vi "NFC_Connect.vi"(9 "VISA resource name":refnum<visa-resource-name>="COM1") -> (1 "NFC":bool, 2 "Response":string)   [LabVIEW 2017]
uses:
  Ctrls/Serial_Settings.ctl
  <vilib>/Instr/_visa.llb/VISA Configure Serial Port (Instr).vi
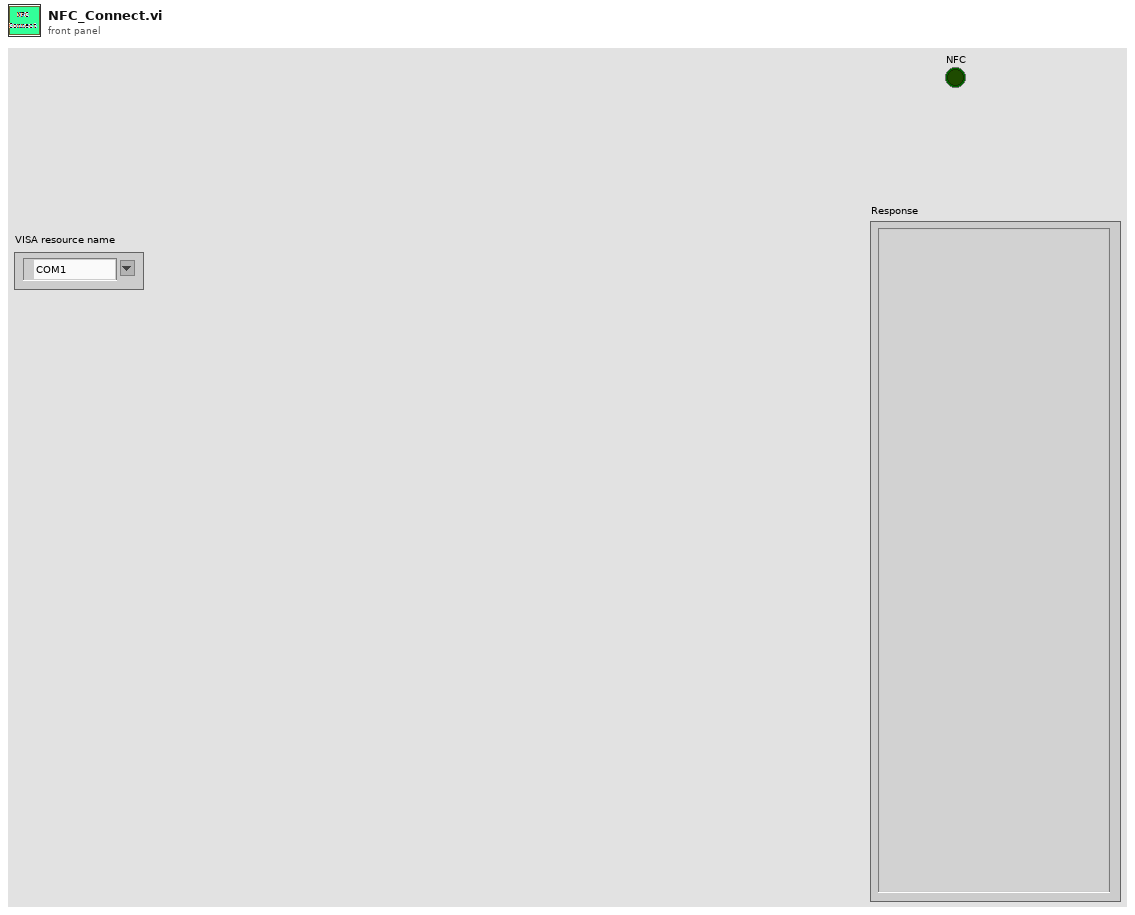
[diagram p1: front panel]
types:
  T1 = typedef "Serial_Settings.ctl" = cluster{"baud rate":u32, "data bits":u16, "parity":enum16{"None", "Odd", "Even", "Mark", "Space"}, "stop bits":u16, "flow control":u16}
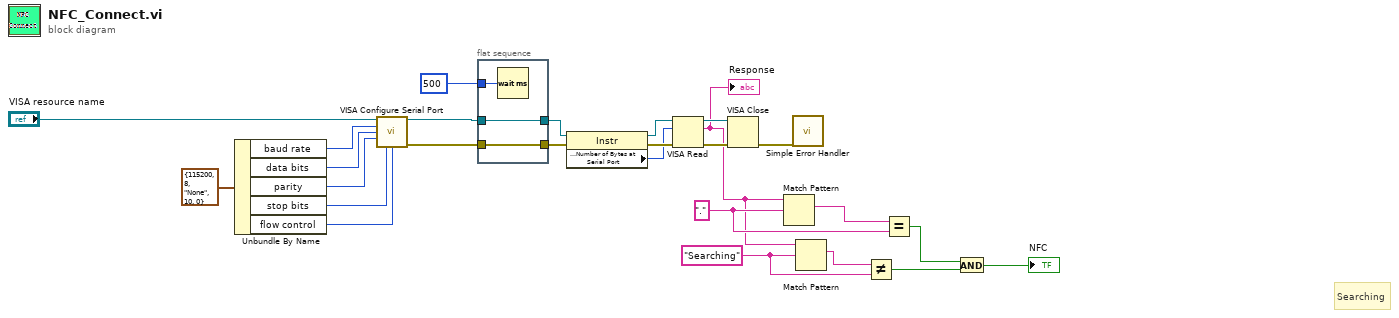
[diagram p0: block diagram]
diagram:
  w4 = "Searching"
  w7 = "."
  # "Searching"
  n1 = Unbundle By Name(T1 {"baud rate"=115200, "data bits"=8, "parity"=enum."None", "stop bits"=10, "flow control"=0} ("Serial Settings")) -> ("baud rate"=w15:u32, "data bits"=w14:u16, "parity"=w13:enum16{"None", "Odd", "Even", "Mark", "Space"}, "stop bits"=w12:u16, "flow control"=w11:u16)
  n2 = call-poly "VISA Configure Serial Port"("VISA resource name"="VISA resource name", "baud rate (9600)"=w15, "data bits (8)"=w14, "parity (0:none)"=w13, "stop bits (10: 1 bit)"=w12, "flow control (0:none)"=w11) -> ("VISA resource name out"=w10:refnum<visa-resource-name>, "error out"=w9:errorcluster)  [unwired: 3 in, 5 out]
  n3 = flat-sequence {
    tunnel: w9 -> [w28]
    tunnel: [w28] -> w22
    tunnel: w10 -> [w27]
    tunnel: [w27] -> w21
    tunnel: u32 500 ("delay before read (ms)") -> [w29]
    frame #0 {
      n4 = Wait (ms)(milliseconds to wait=w29) -> ()  [unwired: 1 out]
    }
  }
  n5 = property class="Instr"(reference=w21, error in=w22) -> (reference out=w19:refnum<visa-resource-name>, error out=w18:errorcluster, "Serial Settings:Number of Bytes at Serial Port"=w17:u32)
  n6 = VISA Read(VISA resource name=w19, byte count=w17, error in (no error)=w18) -> (VISA resource name out=w24:refnum<visa-resource-name>, read buffer=w6:string, error out=w25:errorcluster)  [unwired: 1 out]
  "Response" <- w6
  n7 = VISA Close(VISA resource name=w24, error in (no error)=w25) -> (error out=w23:errorcluster)
  n8 = Match Pattern(string=w6, regular expression=w7) -> (match substring=w8:string)  [unwired: 1 in, 3 out]
  n9 = call <vilib>:"Simple Error Handler.vi"("error in (no error)"=w23) -> ()  [unwired: 1 in, 8 out]
  n10 = Match Pattern(string=w6, regular expression=w4) -> (match substring=w5:string)  [unwired: 1 in, 3 out]
  n11 = Not Equal?(x=w5, y=w4) -> (x != y?=w2:bool)
  n12 = Equal?(x=w8, y=w7) -> (x = y?=w3:bool)
  n13 = And(x=w3, y=w2) -> (x .and. y?=→"NFC":bool)
